vi "tank drive final (1).vi"   [LabVIEW 2010, in "Tank Robot.lvrbt"]
uses:
  Tank Robot.lvrbt
  <vilib>/NXT/Subs/LVHSConnector.ctl
  <vilib>/NXT/NXTIO Xnodes/AddressXNode/NXTIOAddress.xnode
  <vilib>/NXT/Subs/MotorXNode.Servo Type.ctl
  <vilib>/NXT/Subs/MotorXNode.1Servo.ctl
  <vilib>/NXT/NXTIO Xnodes/NXTIOXNode/NXTIO.xnode
  <vilib>/NXT/Subs/MotorXNode.DC Motor Type.ctl
  <vilib>/NXT/Subs/MotorXNode.2DCMotor.ctl
  <vilib>/NXT/NXTIO Xnodes/NXTIONodeSubVIs/TETRIX IO Move Servos.vi
  <vilib>/FTC/FTC Calculate Drive Power - Tank.vi
  <vilib>/NXT/NXTIO Xnodes/NXTIONodeSubVIs/TETRIX IO Move DC Motors.vi
types:
  T1 = typedef "MotorXNode.Servo Type.ctl" = enum16{"Servo"}
  T2 = typedef "FTC ControllerState.ctl" = cluster{"Left X":i8, "Left Y":i8, "Right X":i8, "Right Y":i8, "Button Encoding 9-12":u8, "Button Encoding 1-8":u8, "POV":T3}
  T3 = typedef "FTC POVState.ctl" = i8
  T4 = typedef "MotorXNode.DC Motor Type.ctl" = enum16{"DC Motor"}
  T5 = cluster{"DC Motor":T4, "Address":i16, "Address":i16}
  T6 = typedef "FTC ButtonState.ctl" = cluster{"Button 1":bool, "Button 2":bool, "Button 3":bool, "Button 4":bool, "Button 5":bool, "Button 6":bool, "Button 7":bool, "Button 8":bool, "Button 9":bool, "Button 10":bool, "Button 11":bool, "Button 12":bool, "POV":T3}
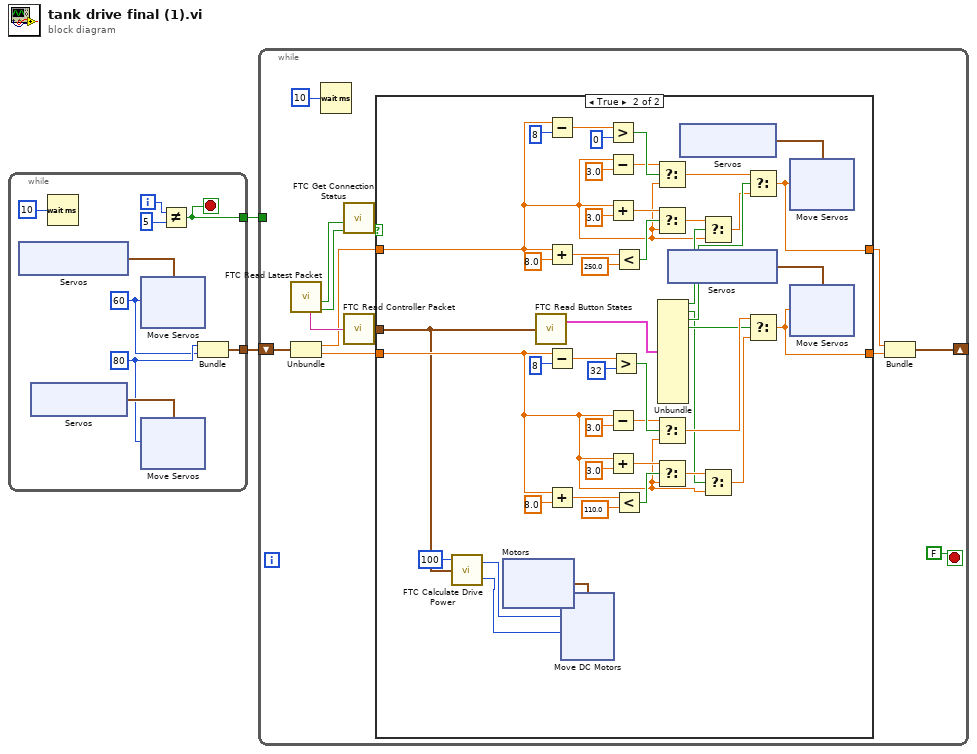
[diagram p0: block diagram]
diagram:
  n1 = while {
    tunnel: [w8] -> w2
    tunnel: [w3] -> w1
    i -> [w11]
    stop <- w8 stop-if-true
    w4 = u8 60 ("Position 1")
    w5 = u8 80 ("Position 1")
    n2 = xnode "Servos"() -> ("Servo"=w6:cluster{"Servo":T1, "Address":i16})
    n3 = xnode "Servos"() -> ("Servo"=w7:cluster{"Servo":T1, "Address":i16})
    n4 = Wait (ms)(milliseconds to wait=u32 10) -> ()  [unwired: 1 out]
    n5 = xnode "Move Servos"("Position 1"=w4, "Servos"=w6) -> ()  [unwired: 1 in, 1 out]
    n6 = xnode "Move Servos"("Position 1"=w5, "Servos"=w7) -> ()  [unwired: 1 in, 1 out]
    n7 = Not Equal?(x=w11, y=5) -> (x != y?=w8:bool)
    n8 = Bundle("Position 1"=w5, "Position 1"=w4) -> (w3:cluster{"Position 1":u8, "Position 1":u8})  [unwired: 1 in]
  }
  n9 = while {
    tunnel: w2 -> [_]
    shift-right: [w30] -> _
    shift-left: w1 -> [w35]
    stop <- FALSE stop-if-true
    n10 = call <vilib>:"FTC Read Latest Packet.vi"() -> ("Packet Received?"=w39:bool, "Stopped?"=w40:bool, "Controller 1"=w37:string)  [unwired: 6 in, 3 out]
    n11 = Unbundle(w35) -> ("Position 1"=w34:dbl, "Position 1"=w33:dbl)
    n12 = Wait (ms)(milliseconds to wait=u32 10) -> ()  [unwired: 1 out]
    n13 = call <vilib>:"FTC Get Connection Status.vi"("Packet Received?"=w39, "Stopped?"=w40) -> ("Online?"=w38:bool)  [unwired: 6 in, 2 out]
    n14 = call <vilib>:"FTC Read Controller Packet.vi"("Packet"=w37) -> ("Controller State"=w36:T2)  [unwired: 4 in]
    n15 = case shown="True" w38 {
      tunnel: w36 -> [_ w49]
      tunnel: w34 -> [w44 w72]
      tunnel: w33 -> [w43 w51]
      tunnel: [w44 w69] -> w32
      tunnel: [w43 w50] -> w31
      frame False {
      }
      frame True {
        n16 = call-poly <vilib>:"FTC Calculate Drive Power.vi"("Controller State"=w49, "Power Level (50)"=i8 100) -> ("Right Motor Power"=w45:i8, "Left Motor Power"=w46:i8)  [unwired: 2 in]
        n17 = xnode "Motors"() -> ("DC Motor"=w47:T5)
        n18 = call <vilib>:"FTC Read Button States.vi"("Controller State"=w49) -> ("Button States"=w90:T6)  [unwired: 2 in, 1 out]
        n19 = Subtract(x=w72, y=u8 8) -> (x-y=w87:dbl)
        n20 = Add(x=w72, y=8.0) -> (x+y=w78:dbl)
        n21 = Subtract(x=w51, y=u8 8) -> (x-y=w67:dbl)
        n22 = Add(x=w51, y=8.0) -> (x+y=w60:dbl)
        n23 = xnode "Move DC Motors"("Power/Speed 2"=w45, "Power/Speed 1"=w46, "Motors"=w47) -> ()  [unwired: 1 in, 1 out]
        n24 = Greater?(x=w87, y=u8 0) -> (0:w85:bool)
        n25 = Subtract(x=w72, y=3.0) -> (x-y=w84:dbl)
        n26 = Add(x=w72, y=3.0) -> (x+y=w75:dbl)
        n27 = Subtract(x=w51, y=3.0) -> (x-y=w64:dbl)
        n28 = Add(x=w51, y=3.0) -> (x+y=w57:dbl)
        n29 = Greater?(x=w67, y=u8 32) -> (0:w65:bool)
        n30 = Less?(x=w78, y=250.0) -> (x < y?=w76:bool)
        n31 = Less?(x=w60, y=110.0) -> (x < y?=w58:bool)
        n32 = Select(t=w84, s=w85, f=w72) -> (s? t:f=w82:dbl)
        n33 = Select(t=w75, s=w76, f=w72) -> (s? t:f=w73:dbl)
        n34 = Select(t=w64, s=w65, f=w51) -> (s? t:f=w62:dbl)
        n35 = Select(t=w57, s=w58, f=w51) -> (s? t:f=w55:dbl)
        n36 = Unbundle(w90) -> ("Button 1"=w80:bool, "Button 2"=w52:bool, "Button 3"=w81:bool, "Button 4"=w53:bool)  [unwired: 9 out]
        n37 = xnode "Servos"() -> ("Servo"=w70:cluster{"Servo":T1, "Address":i16})
        n38 = xnode "Servos"() -> ("Servo"=w89:cluster{"Servo":T1, "Address":i16})
        n39 = Select(t=w73, s=w80, f=w72) -> (s? t:f=w71:dbl)
        n40 = Select(t=w55, s=w52, f=w51) -> (s? t:f=w54:dbl)
        n41 = Select(t=w82, s=w81, f=w71) -> (s? t:f=w69:dbl)
        n42 = Select(t=w62, s=w53, f=w54) -> (s? t:f=w50:dbl)
        n43 = xnode "Move Servos"("Position 1"=w69, "Servos"=w89) -> ()  [unwired: 1 in, 1 out]
        n44 = xnode "Move Servos"("Position 1"=w50, "Servos"=w70) -> ()  [unwired: 1 in, 1 out]
      }
    }
    n45 = Bundle("Position 1"=w32, "Position 1"=w31) -> (w30:cluster{"Position 1":dbl, "Position 1":dbl})  [unwired: 1 in]
  }
